vi "Window1.vi"() -> ()   [LabVIEW 8.6]
uses:
  user32.dll
  EventHandlerEnum.ctl
panel:
  in  "Tab Control":enum32{"Main", "Setup", "Debug Data"}(tab)
  out "?":sgl(knob) scale=-5.0..5.0 scale format="%#.2g"
  out "Course/Bearing":cluster{i16, i16}(knob) scale=0.0..360.0 scale format="%.0f°"
  out "Altitude":cluster{i32, i32}(knob) scale=0.0..200.0
  out "Air Speed":cluster{i16, i16}(knob)={0, 31} scale=0.0..40.0
  out "UAV Longitude 2":dbl format="%.6g°"
  out "Est Time Left":i32
  out "Current WP":i32
  out "Amps":i32
  out "Watts":i32
  out "Throttle":dbl(slide) scale=0.0..100.0
  out "Battery":dbl(slide) scale=0.0..10.0
  out "Pitch":i32
  out "Roll":i32
  out "Nav Display":picture
  out "Distance to WP":i32 format="%.0f m"
  out "Ground Speed":i32 format="%.0f m/s"
  out "Air Speed":i32 format="%.0f m/s"
  out "UAV Longitude":dbl format="%.6g°"
  out "UAV Latitude":dbl format="%.6g°"
  in  "Stop":bool
  in  "WebBrowser":refnum<k7>(container)
  out "StreamingProgressPercentage":i32(slide) scale=0.0..100.0
  in  "Baud Rate":string(combo)="9600"
  in  "Choose Port":refnum<visa-resource-name>="COM1"
  out "Camera Position 2":T1
  out "Version":string
  out "VersionAppType":i32(ring) items=["EnterpriseClientGE", "ProGE", "PlusGE", "FreeGE", "UnknownGE"]
  out "ElevationExaggeration":dbl
  in  "Set":bool
  in  "AutoPilotSpeed":dbl=0.5
  in  "error in":errorcluster
  in  "EARTHLib.IApplicationGE 2":refnum<k7>
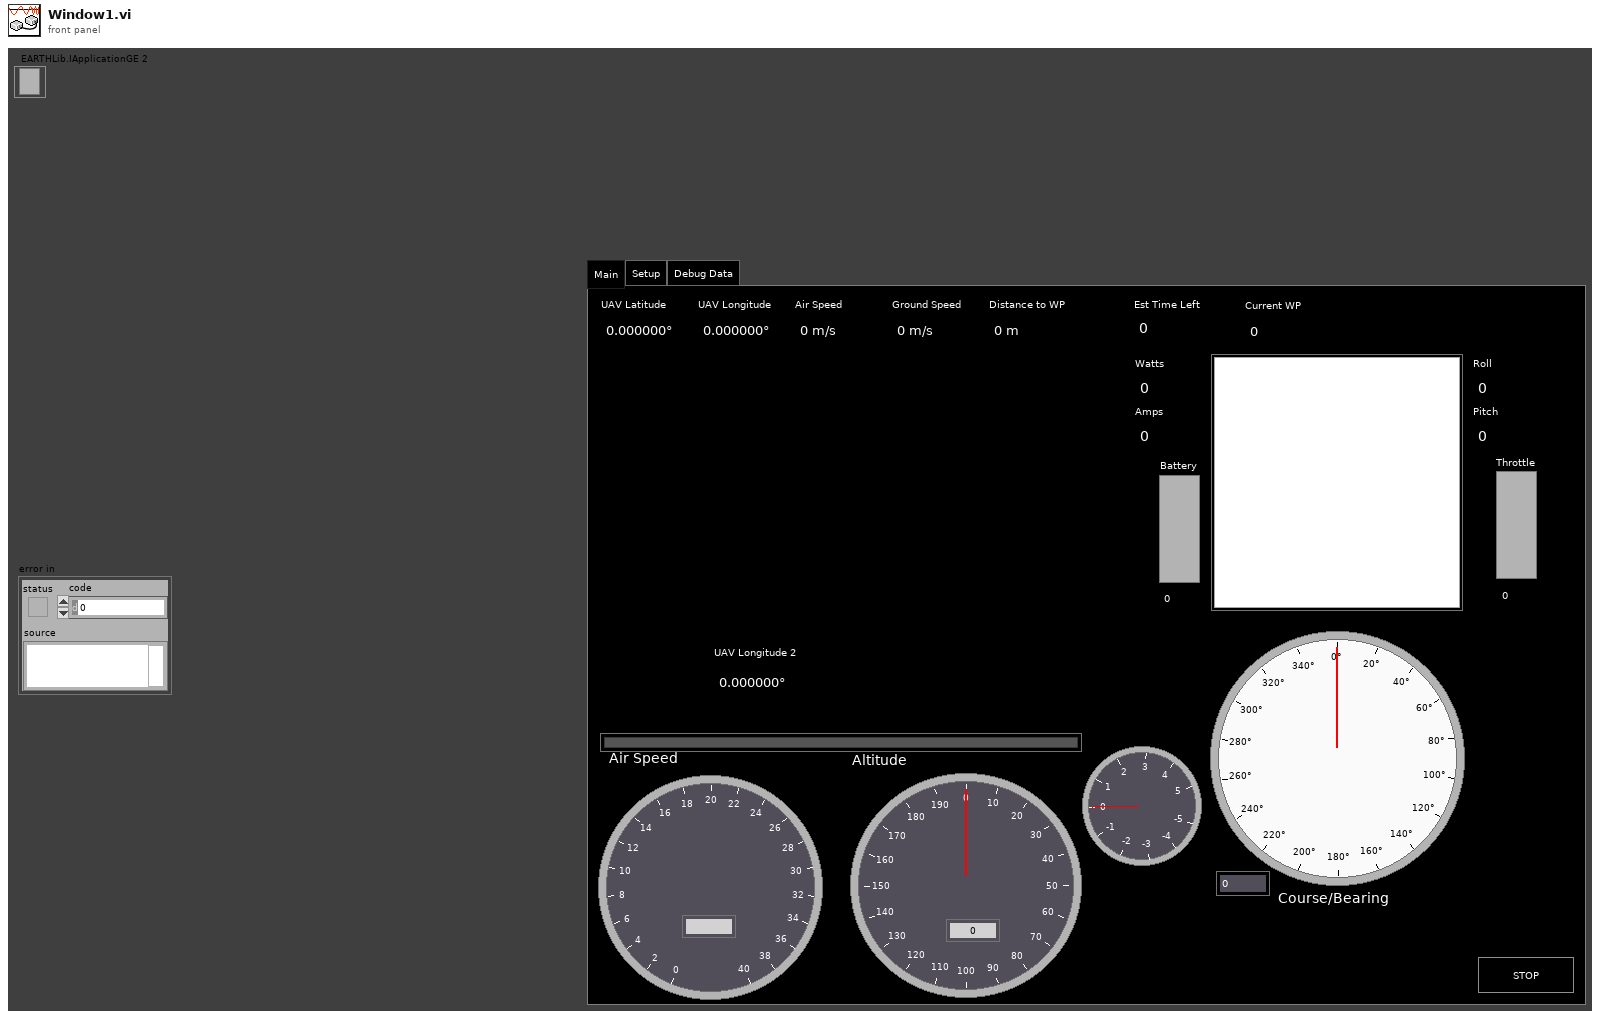
[diagram p1: front panel]
types:
  T1 = cluster{"Azimuth":dbl, "FocusPointAltitude":dbl, "FocusPointAltitudeMode":i32, "FocusPointLatitude":dbl, "FocusPointLongitude":dbl, "Range":dbl, "Tilt":dbl}
  T2 = typedef "EventHandlerEnum.ctl" = enum16{"Timeout", "Stop"}
  T3 = typedef "imagedata.ctl" = cluster{"image type":i32, "image depth":i32, "image":u8[], "mask":u8[], "colors":u32[], "Rectangle":cluster{"left":i16, "top":i16, "right":i16, "bottom":i16}}
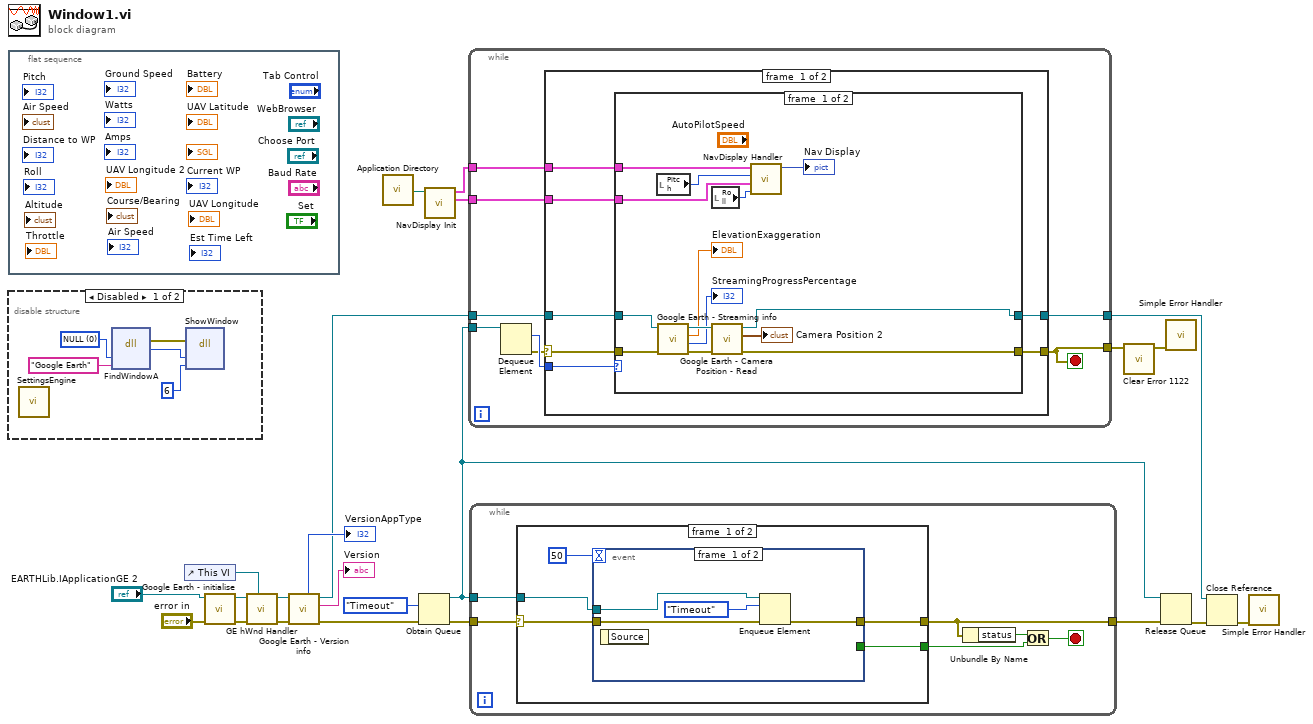
[diagram p0: block diagram]
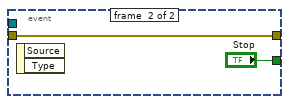
[diagram p4: hidden frame]
diagram:
  n1 = flat-sequence {
    frame #0 {
    }
  }
  n2 = disable-structure shown="Disabled" {
    frame #0 {
      w28 = 0 items=["NULL"]
      n3 = call "SettingsEngine.vi"() -> ()  [unwired: 10 in, 2 out]
      n4 = dll-call lib="user32.dll" fn="FindWindowA" label="FindWindow"("lpszClassName"=w28, "lpszWindowName"="Google Earth") -> (error out=w27:errorcluster, "hWnd"=w25:u32)  [unwired: 4 in, 2 out]
      n5 = dll-call lib="user32.dll" fn="ShowWindow"(error in=w27, "hWnd"=w25, "nCmdShow"=u32 6) -> ()  [unwired: 3 in, 4 out]
    }
    frame #1 {
    }
  }
  n6 = control-ref of="This VI"() -> (w19:refnum<vi>)
  n7 = call "Google Earth - initialise.vi"("error in (no error)"="error in", "EARTHLib.IApplicationGE"="EARTHLib.IApplicationGE 2") -> ("error out"=w11:errorcluster, "Refnum Out"=w10:refnum<k7>)  [unwired: 7 in, 1 out]
  n8 = call "GE hWnd Handler.vi"("This VI"=w19, "error in"=w11, "Refnum In"=w10) -> ("error out"=w20:errorcluster, "Refnum Out"=w12:refnum<k7>)  [unwired: 7 in]
  n9 = call "Google Earth - Version info.vi"("error in"=w20, "Refnum In"=w12) -> ("error out"=w17:errorcluster, "Version"=→"Version":string, "Refnum Out"=w16:refnum<k7>, "VersionAppType"=→"VersionAppType":i32)  [unwired: 6 in]
  n10 = call <vilib>:"Application Directory.vi"() -> ("Application Directory"=w9:path)
  n11 = Obtain Queue(element data type=EventHandlerEnum."Timeout" ("Enum"), error in (no error)=w17) -> (queue out=w21:refnum<queue>, error out=w1:errorcluster)  [unwired: 3 in, 1 out]
  n12 = call "NavDisplay Init.vi"("Application Directory"=w9) -> ("roll image"=w8:T3, "pitch image"=w7:T3)  [unwired: 8 in]
  n13 = while {
    tunnel: w21 -> [w36]
    tunnel: [w29] -> w4
    tunnel: w16 -> [w34]
    tunnel: [w33] -> w13
    tunnel: w8 -> [w31]
    tunnel: w7 -> [w30]
    stop <- w29 stop-if-true
    n14 = Dequeue Element(queue=w36) -> (element=w35:T2, error out=w32:errorcluster)  [unwired: 2 in, 2 out]
    n15 = case shown="No Error" w32 {
      selector: w32 -> [w41 w61]
      tunnel: w35 -> [w43 _]
      tunnel: w34 -> [w42 w60]
      tunnel: [w40 w61] -> w29
      tunnel: [w39 w60] -> w33
      tunnel: w30 -> [w38 _]
      tunnel: w31 -> [w37 _]
      frame #0 {
        n16 = case shown="\"Timeout\", Default" w43 {
          tunnel: w42 -> [w52 w59]
          tunnel: w41 -> [w51 w58]
          tunnel: [w44 w58] -> w40
          tunnel: [w45 w59] -> w39
          tunnel: w38 -> [w47 _]
          tunnel: w37 -> [w46 _]
          frame #0 {
            n17 = local read "Pitch"() -> (w49:i32)
            n18 = call "Google Earth - Streaming info.vi"("error in"=w51, "Refnum in"=w52) -> ("error out"=w57:errorcluster, "StreamingProgressPercentage"=→"StreamingProgressPercentage":i32, "ElevationExaggeration"=→"ElevationExaggeration":dbl, "Refnum Out"=w56:refnum<k7>)  [unwired: 5 in, 1 out]
            n19 = local read "Roll"() -> (w50:i32)
            n20 = call "Google Earth - Camera Position - Read.vi"("error in"=w57, "Refnum in"=w56) -> ("error out"=w44:errorcluster, "Camera Position"=→"Camera Position 2":T1, "Refnum Out"=w45:refnum<k7>)  [unwired: 7 in]
            n21 = call "NavDisplay Handler.vi"("Roll"=w50, "roll image"=w46, "Pitch"=w49, "pitch image"=w47) -> ("new picture"=→"Nav Display":picture)  [unwired: 6 in]
          }
          frame #1 {
            # "Reset controls to default, or animate sliders back to 0"
          }
        }
      }
      frame #1 {
      }
    }
  }
  n22 = while {
    tunnel: w21 -> [w67]
    tunnel: w1 -> [w62]
    tunnel: [w65] -> w6
    stop <- w63 stop-if-true
    n23 = case shown="No Error" w62 {
      selector: w62 -> [w68 w79]
      tunnel: w67 -> [w72 _]
      tunnel: [w70 w79] -> w65
      tunnel: [w69 _] -> w64
      frame #0 {
        n24 = event shown="[1] \"Stop\": Value Change" {
          selector: _ -> [_ _]
          dyn-events: _ -> [_ _]
          timeout: 50 -> [_ _]
          tunnel: w72 -> [w76 _]
          tunnel: w68 -> [w75 w77]
          tunnel: [w74 w77] -> w70
          tunnel: [_ "Stop"] -> w69
          event #0 {
            n25 = event-data() -> ()  [unwired: 1 in, 1 out]
            n26 = Enqueue Element(queue=w76, element=EventHandlerEnum."Timeout", error in (no error)=w75) -> (error out=w74:errorcluster)  [unwired: 1 in, 2 out]
          }
          event #1 {
            n27 = event-data() -> ()  [unwired: 1 in, 2 out]
          }
        }
      }
      frame #1 {
      }
    }
    n28 = Unbundle By Name(w65) -> ("status"=w66:bool)
    n29 = Or(x=w66, y=w64) -> (x .or. y?=w63:bool)
  }
  n30 = call "Clear Error 1122.vi"("error in"=w4) -> ("error out"=w3:errorcluster)  [unwired: 10 in]
  n31 = Release Queue(queue=w21, error in (no error)=w6) -> (error out=w2:errorcluster)  [unwired: 1 in, 2 out]
  n32 = call <vilib>:"Simple Error Handler.vi"("error in (no error)"=w3) -> ()  [unwired: 4 in, 5 out]
  n33 = Close Reference(reference=w13, error in (no error)=w2) -> (error out=w5:errorcluster)
  n34 = call <vilib>:"Simple Error Handler.vi"("error in (no error)"=w5) -> ()  [unwired: 4 in, 5 out]
